vi "HostExample.vi"() -> ()   [LabVIEW 2023]
uses:
  deps/hdl-shared/host_interfaces/fifo/LabVIEW/HdlFifo/NiFpga_HdlFifo_WriteI32.vi
  deps/hdl-shared/host_interfaces/fifo/LabVIEW/HdlFifo/NiFpga_HdlFifo_ReadI32.vi
  <vilib>/FPGAPlugInAG/Dynamic/niLvFpga_Download_Dynamic.vi
  <vilib>/FPGAPlugInAG/Dynamic/niLvFpga_Run_Dynamic.vi
  deps/hdl-shared/host_interfaces/fifo/LabVIEW/HdlFifo/NiFpga_HdlFifo_AddI32.vi
  deps/hdl-shared/host_interfaces/fifo/LabVIEW/HdlFifo/private/_NiFpga_HdlFifo_GetStream.vi
  <vilib>/Utility/error.llb/Error Cluster From Error Code.vi
  <vilib>/rvi/interface/nirviMethod/nirviMethod.xnode
panel:
  in  "Device address":string="PXI1Slot2"
  in  "Bitfile path":path=path "C:/dev/github20-test/flexrio-custom/targets/pxie-7912custom/docs/Examples/LV2023/BlankRunningVI/FPGA Bitfiles/blankrunningvi_FPGATarget_BlankRunningVI2_1nxfS5+mbi0.lvbitx"
  out "empty elements remaining":u64
  out "Elements Remaining":u64
  out "error out":errorcluster
  in  "WriteScratch":bool
  in  "ReadScratch":bool
  out "Scratch Read":u32 format="%.0x"
  in  "Scratch Write":u32 format="%.0x"
  in  "Num Elements":i32
  out "Read Data":u32[](array[numeric])
  in  "Read FPGA FIFO":bool
  in  "Write FPGA FIFO":bool
  in  "Write Data":u32[](array[numeric])
  in  "WriteReg":bool
  in  "ReadReg":bool
  out "Read Value":u32
  in  "Write Value":u32 format="%.0x"
  in  "Write Offset":u32
  in  "Read Offset":u32
  in  "Num Elements":i32
  out "Data 4":i32[](array[numeric])
  in  "Write Data":i32[](array[numeric])
  in  "Read Host FIFO":bool
  in  "Write Host FIFO":bool
  out "Numeric":i32
  in  "stop":bool
  # "Write and read any register offset"
  # "Write and read the scratch register"
  # "Scratch Register"
  # "Write and read the Host to FPGA FIFO"
  # "Host to FPGA FIFO"
  # "Write and read the FPGA to Host FIFO"
  # "FPGA to Host FIFO"
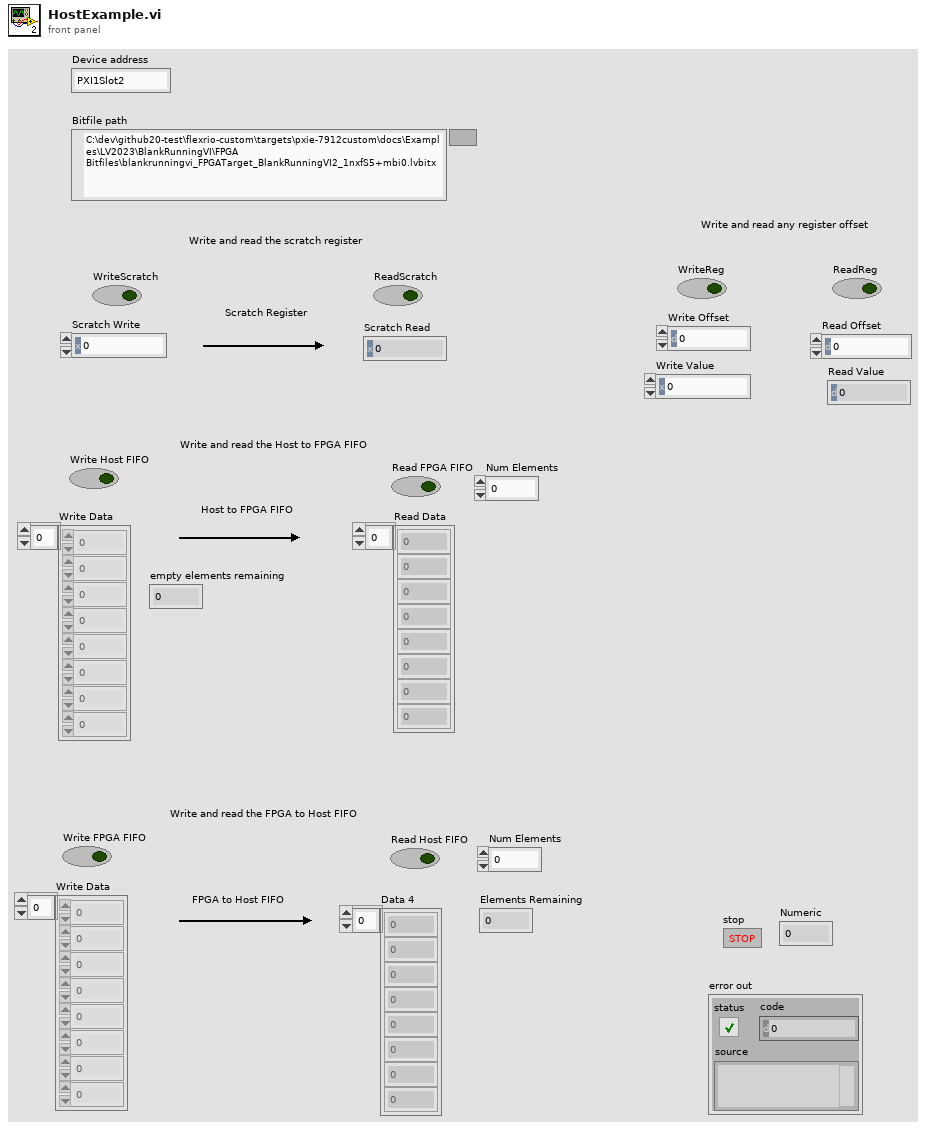
[diagram p1: front panel]
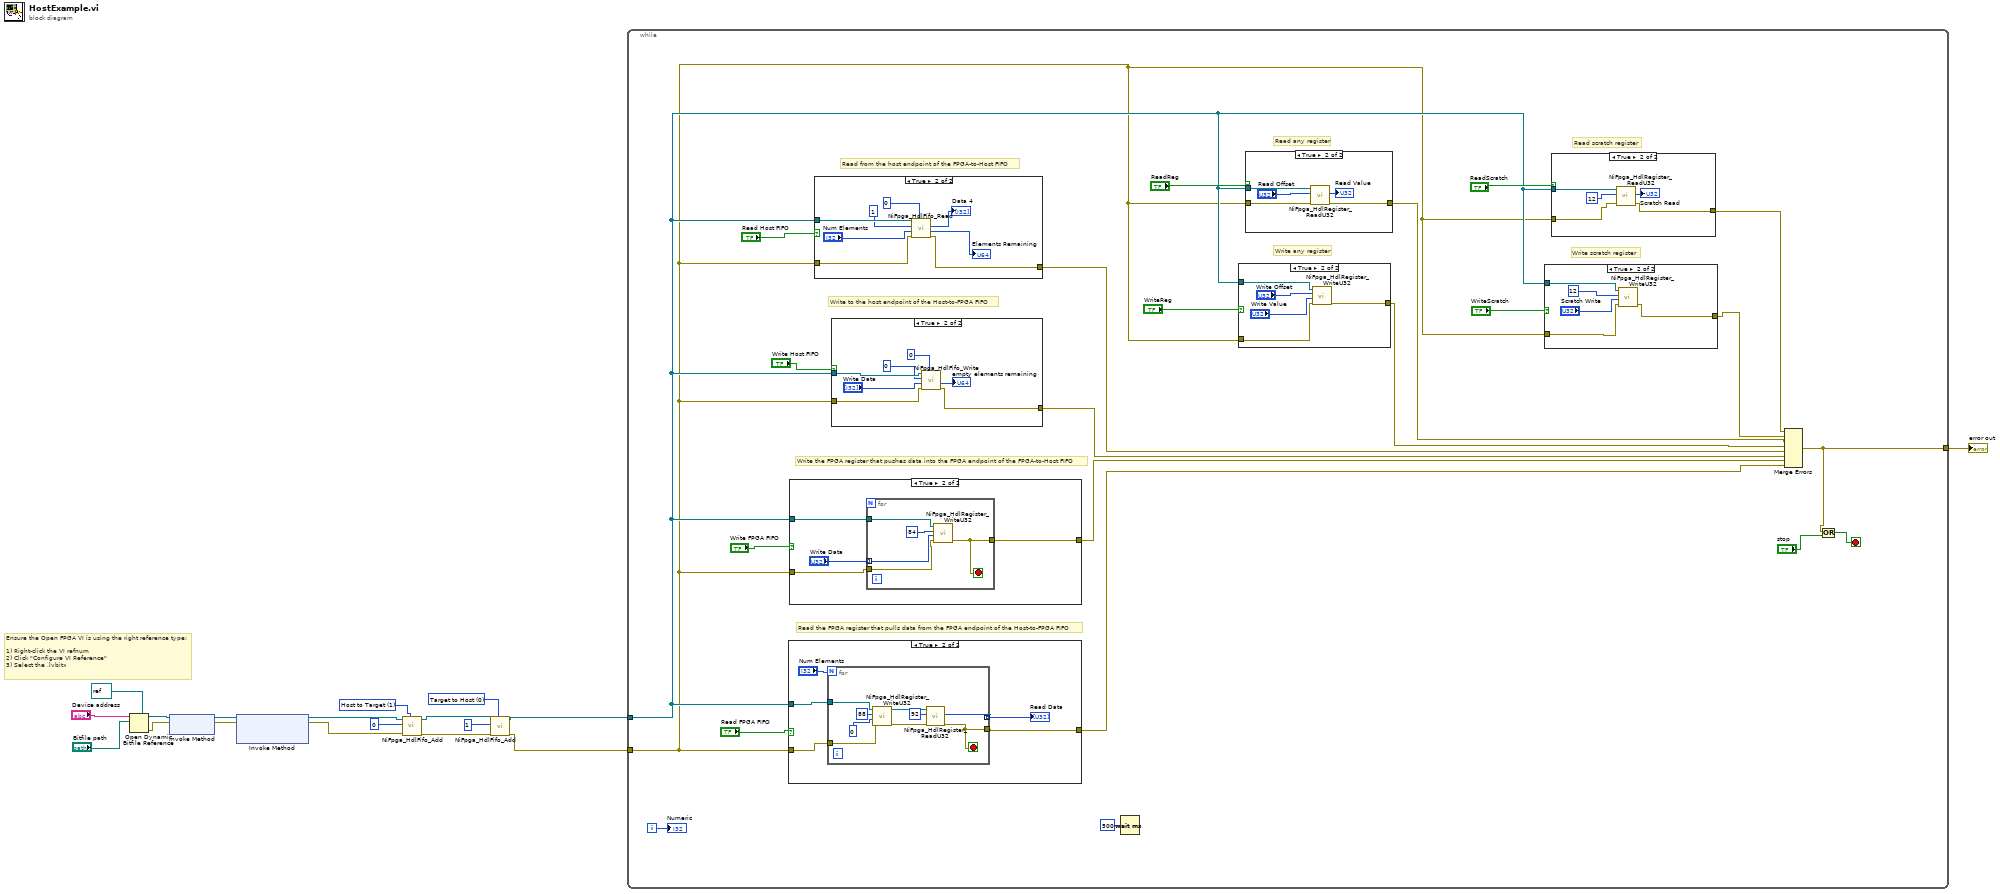
[diagram p0: block diagram]
diagram:
  w4 = u32 0 items=["Target to Host", "Host to Target"] ("direction")
  w10 = u32 1 items=["Target to Host", "Host to Target"]
  # "Ensure the Open FPGA VI is using the right reference type:\n\n1) Right-click the VI refnum \n2) Click \"Configure VI Reference\"\n3) Select the .lvbitx"
  n1 = Open Dynamic Bitfile Reference(0:"Device address", 1:"Bitfile path", 4:refnum<k20> refnum ("Type")) -> (5:w15:refnum<k20>, 8:w14:errorcluster)  [unwired: 2 in]
  n2 = xnode "Invoke Method"("FPGA VI Reference In"=w15, "error in"=w14) -> ("FPGA VI Reference Out"=w17:refnum<k20>, "error out"=w18:errorcluster)
  n3 = xnode "Invoke Method"("FPGA VI Reference In"=w17, "error in"=w18) -> ("FPGA VI Reference Out"=w11:refnum<k20>, "error out"=w5:errorcluster)  [unwired: 1 in]
  n4 = call-poly "NiFpga_HdlFifo_Add.vi"("direction"=w10, "error in (no error)"=w5, "Fifo Number"=u32 0, "FPGA VI Reference In"=w11) -> ("error out"=w3:errorcluster, "FPGA VI Reference Out"=w7:refnum<k20>)  [unwired: 6 in]
  n5 = call-poly "NiFpga_HdlFifo_Add.vi"("direction"=w4, "error in (no error)"=w3, "Fifo Number"=u32 1, "FPGA VI Reference In"=w7) -> ("error out"=w2:errorcluster, "FPGA VI Reference Out"=w8:refnum<k20>)  [unwired: 6 in]
  n6 = while {
    tunnel: w8 -> [w31]
    tunnel: w2 -> [w30]
    tunnel: [w19] -> w1
    i -> [w41]
    stop <- w21 stop-if-true
    # "Write scratch register"
    # "Read scratch register"
    # "Read any register"
    # "Write any register"
    # "Read from the host endpoint of the FPGA-to-Host FIFO"
    # "Write to the host endpoint of the Host-to-FPGA FIFO"
    # "Read the FPGA register that pulls data from the FPGA endpoint of the Host-to-FPGA FIFO"
    # "Write the FPGA register that pushes data into the FPGA endpoint of the FPGA-to-Host FIFO"
    n7 = case shown="True" "Read FPGA FIFO" {
      tunnel: w31 -> [_ w59]
      tunnel: w30 -> [w54 w56]
      tunnel: [w54 w55] -> w22
      frame False {
      }
      frame True {
        n8 = for {
          N: "Num Elements" -> [_]
          tunnel: w59 -> [w68]
          tunnel: [w64] -> w58 mode=indexing
          tunnel: w56 -> [w62]
          tunnel: [w60] -> w55
          stop <- w60 stop-if-true
          n9 = call "NiFpga_HdlRegister_WriteU32.vi"("error in (no error)"=w62, "Value"=u32 0, "Offset"=u32 88, "FPGA VI Reference In"=w68) -> ("error out"=w61:errorcluster, "FPGA VI Reference Out"=w66:refnum<k20>)  [unwired: 5 in]
          n10 = call "NiFpga_HdlRegister_ReadU32.vi"("error in (no error)"=w61, "Offset"=u32 92, "FPGA VI Reference In"=w66) -> ("error out"=w60:errorcluster, "Value"=w64:u32)  [unwired: 6 in, 1 out]
        }
        "Read Data" <- w58
      }
    }
    n11 = case shown="True" "Write FPGA FIFO" {
      tunnel: w31 -> [_ w73]
      tunnel: w30 -> [w69 w71]
      tunnel: [w69 w70] -> w23
      frame False {
      }
      frame True {
        n12 = for {
          tunnel: w73 -> [w78]
          tunnel: "Write Data" -> [w76] mode=indexing
          tunnel: w71 -> [w75]
          tunnel: [w74] -> w70
          stop <- w74 stop-if-true
          n13 = call "NiFpga_HdlRegister_WriteU32.vi"("error in (no error)"=w75, "Value"=w76, "Offset"=u32 84, "FPGA VI Reference In"=w78) -> ("error out"=w74:errorcluster)  [unwired: 5 in, 1 out]
        }
      }
    }
    n14 = case shown="True" "Read Host FIFO" {
      tunnel: w31 -> [_ w106]
      tunnel: w30 -> [w99 w101]
      tunnel: [w99 w100] -> w25
      frame False {
      }
      frame True {
        n15 = call-poly "NiFpga_HdlFifo_Read.vi"("timeout"=u32 0, "error in (no error)"=w101, "number of elements"="Num Elements", "fifo number"=u32 1 ("Fifo Number"), "fpga vi reference in"=w106) -> ("error out"=w100:errorcluster, "elements remaining"=→"Elements Remaining":u64, "data out"=→"Data 4":i32[])  [unwired: 2 in, 1 out]
      }
    }
    n16 = case shown="True" "Write Host FIFO" {
      tunnel: w31 -> [_ w97]
      tunnel: w30 -> [w91 w93]
      tunnel: [w91 w92] -> w24
      frame False {
      }
      frame True {
        n17 = call-poly "NiFpga_HdlFifo_Write.vi"("timeout"=u32 0, "error in (no error)"=w93, "data in"="Write Data", "fifo number"=u32 0 ("Fifo Number 2"), "fpga vi reference in"=w97) -> ("error out"=w92:errorcluster, "empty elements remaining"=→"empty elements remaining":u64)  [unwired: 3 in, 1 out]
      }
    }
    n18 = Wait (ms)(milliseconds to wait=u32 500) -> ()  [unwired: 1 out]
    n19 = case shown="True" "WriteReg" {
      tunnel: w31 -> [_ w84]
      tunnel: w30 -> [w79 w81]
      tunnel: [w79 w80] -> w26
      frame False {
      }
      frame True {
        n20 = call "NiFpga_HdlRegister_WriteU32.vi"("error in (no error)"=w81, "Value"="Write Value", "Offset"="Write Offset", "FPGA VI Reference In"=w84) -> ("error out"=w80:errorcluster)  [unwired: 5 in, 1 out]
      }
    }
    n21 = case shown="True" "ReadReg" {
      tunnel: w31 -> [_ w90]
      tunnel: w30 -> [w85 w87]
      tunnel: [w85 w86] -> w27
      frame False {
      }
      frame True {
        n22 = call "NiFpga_HdlRegister_ReadU32.vi"("error in (no error)"=w87, "Offset"="Read Offset", "FPGA VI Reference In"=w90) -> ("error out"=w86:errorcluster, "Value"=→"Read Value":u32)  [unwired: 6 in, 1 out]
      }
    }
    n23 = case shown="True" "WriteScratch" {
      tunnel: w31 -> [_ w47]
      tunnel: w30 -> [w42 w44]
      tunnel: [w42 w43] -> w28
      frame False {
      }
      frame True {
        n24 = call "NiFpga_HdlRegister_WriteU32.vi"("error in (no error)"=w44, "Value"="Scratch Write", "Offset"=u32 12 ("Write Offset 2"), "FPGA VI Reference In"=w47) -> ("error out"=w43:errorcluster)  [unwired: 5 in, 1 out]
      }
    }
    n25 = case shown="True" "ReadScratch" {
      tunnel: w31 -> [_ w53]
      tunnel: w30 -> [w48 w50]
      tunnel: [w48 w49] -> w29
      frame False {
      }
      frame True {
        n26 = call "NiFpga_HdlRegister_ReadU32.vi"("error in (no error)"=w50, "Offset"=u32 12 ("Read Offset 2"), "FPGA VI Reference In"=w53) -> ("error out"=w49:errorcluster, "Value"=→"Scratch Read":u32)  [unwired: 6 in, 1 out]
      }
    }
    n27 = Merge Errors(w29, w28, w27, w26, w25, w24, w23, w22) -> (w19:errorcluster)
    n28 = Or(x=w19, y="stop") -> (x .or. y?=w21:bool)
    "Numeric" <- w41
  }
  "error out" <- w1
